vi "Git-Enterprise-Get All Repos In Org.vi"(8 "Error In":errorcluster, 9 "Organization":string, 10 "Server":string, 11 "Refnum in":T2) -> (0 "Error out":errorcluster, 3 "Repos":T1[](array[typedef]))   [LabVIEW 2020]
uses:
  <vilib>/httpClient/ClientHandle.ctl
  Git-Repo JSON Typedef.ctl
  <vilib>/JDP Science/JSONtext/String Subset.vi
  <vilib>/JDP Science/JSONtext/Parsing/Parse Full Path or Item Name.vi
  <vilib>/JDP Science/JSONtext/Offset/Find Item Locations by Path.vi
  <vilib>/httpClient/LabVIEWHTTPClient.lvlib
  <vilib>/JDP Science/JSONtext/JSONtext.lvlib
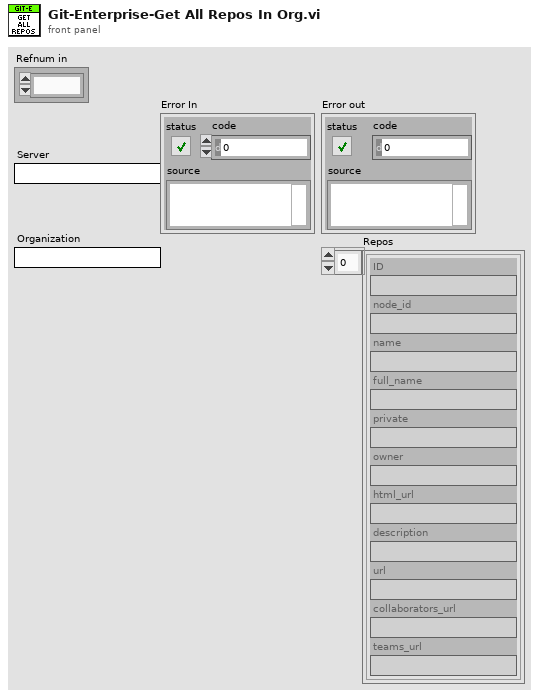
[diagram p1: front panel]
types:
  T1 = typedef "Git-Repo JSON Typedef.ctl" = cluster{"ID":string, "node_id":string, "name":string, "full_name":string, "private":string, "owner":string, "html_url":string, "description":string, "url":string, "collaborators_url":string, "teams_url":string}
  T2 = typedef "LabVIEWHTTPClient.lvlib/ClientHandle.ctl" = refnum<k1>
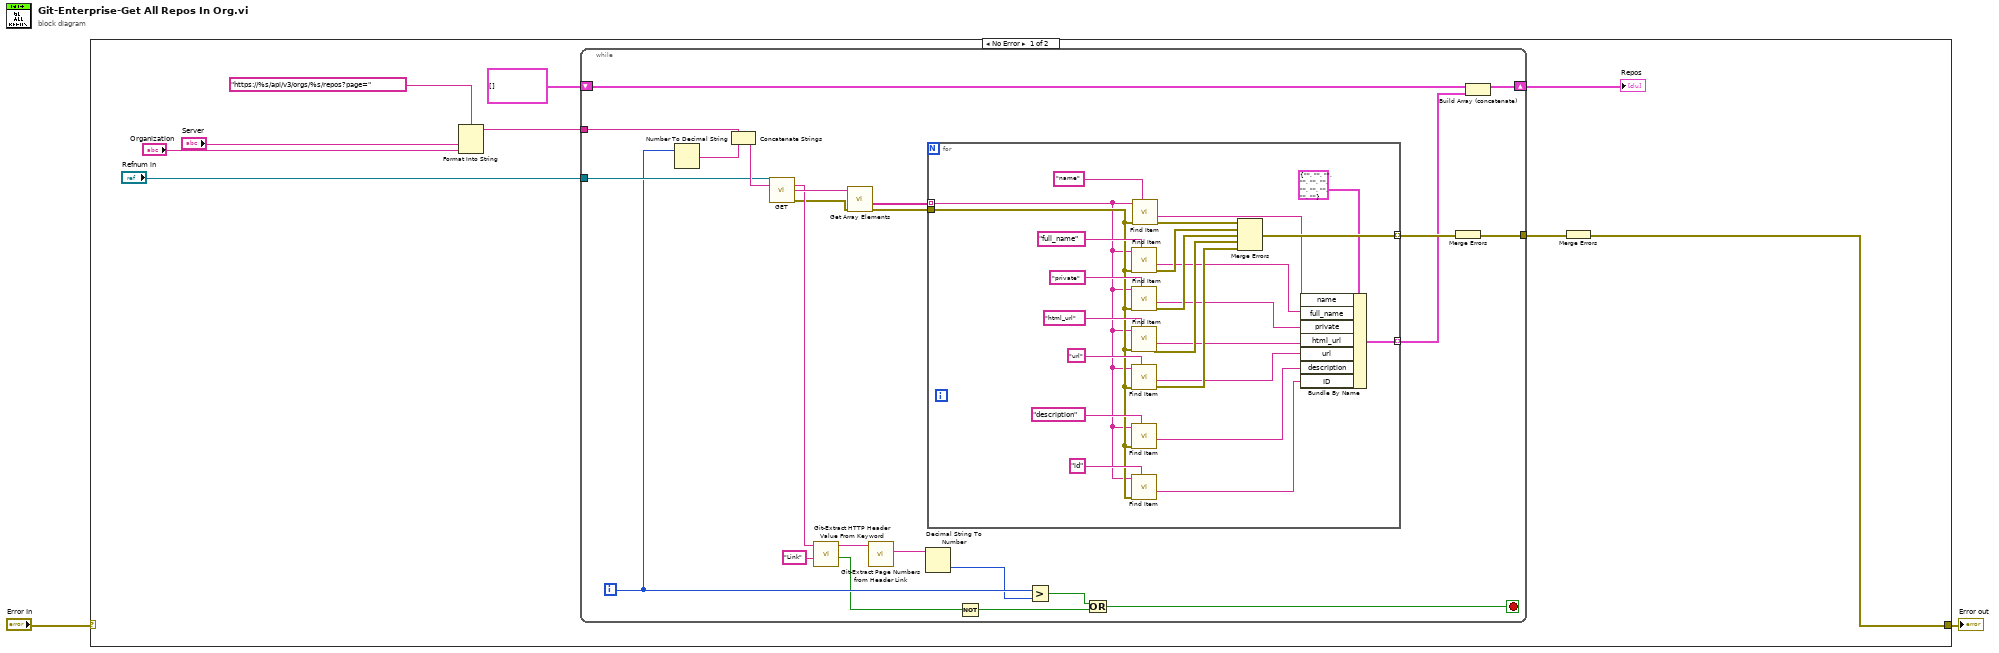
[diagram p0: block diagram]
diagram:
  n1 = case shown="No Error" "Error In" {
    selector: "Error In" -> [_ w59]
    tunnel: [w4 w59] -> w1
    frame No Error {
      n2 = Format Into String(format string="https://%s/api/v3/orgs/%s/repos?page=" ("url"), "Server", "Organization") -> (resulting string=w11:string)  [unwired: 2 in, 1 out]
      n3 = while {
        tunnel: "Refnum in" -> [w33]
        shift-right: [w29] -> w3
        shift-left: T1[] [] -> [w30]
        tunnel: w11 -> [w20]
        tunnel: [w18] -> w5
        i -> [w32]
        stop <- w13 stop-if-true
        n4 = Number To Decimal String(number=w32) -> (decimal integer string=w31:string)  [unwired: 1 in]
        n5 = Concatenate Strings(w20, w31) -> (w34:string)
        n6 = call <vilib>:"GET.vi"("client handle"=w33, "url"=w34) -> ("headers"=w22:string, "body"=w26:string, "error out"=w17:errorcluster)  [unwired: 10 in, 1 out]
        n7 = call "Git-Extract HTTP Header Value From Keyword.vi"("Key"="Link", "Header Info"=w22) -> ("Found"=w15:bool, "Value"=w23:string)  [unwired: 8 in]
        n8 = call <vilib>:"Get Array Elements.vi"("error in (no error)"=w17, "JSON"=w26) -> ("error out"=w28:errorcluster, "<JSON>"=w27:string[])  [unwired: 7 in, 1 out]
        n9 = call "Git-Extract Page Numbers from Header Link.vi"("Link"=w23) -> ("Pages"=w25:string)  [unwired: 9 in, 1 out]
        n10 = Decimal String To Number(string=w25) -> (number=w21:i32)  [unwired: 2 in, 1 out]
        n11 = for {
          tunnel: w27 -> [w36] mode=indexing
          tunnel: w28 -> [w37]
          tunnel: [w48] -> w19 mode=indexing
          tunnel: [w39] -> w12 mode=indexing
          n12 = call <vilib>:"Find Item.vi"("$Path or Item Name"="full_name", "error in (no error)"=w37, "JSON"=w36) -> ("error out"=w52:errorcluster, "<JSON>"=w45:string)  [unwired: 5 in, 2 out]
          n13 = call <vilib>:"Find Item.vi"("$Path or Item Name"="private", "error in (no error)"=w37, "JSON"=w36) -> ("error out"=w51:errorcluster, "<JSON>"=w44:string)  [unwired: 5 in, 2 out]
          n14 = call <vilib>:"Find Item.vi"("$Path or Item Name"="html_url", "error in (no error)"=w37, "JSON"=w36) -> ("error out"=w50:errorcluster, "<JSON>"=w43:string)  [unwired: 5 in, 2 out]
          n15 = call <vilib>:"Find Item.vi"("$Path or Item Name"="url", "error in (no error)"=w37, "JSON"=w36) -> ("error out"=w49:errorcluster, "<JSON>"=w42:string)  [unwired: 5 in, 2 out]
          n16 = call <vilib>:"Find Item.vi"("$Path or Item Name"="description", "error in (no error)"=w37, "JSON"=w36) -> ("<JSON>"=w40:string)  [unwired: 5 in, 3 out]
          n17 = call <vilib>:"Find Item.vi"("$Path or Item Name"="id", "error in (no error)"=w37, "JSON"=w36) -> ("<JSON>"=w35:string)  [unwired: 5 in, 3 out]
          n18 = call <vilib>:"Find Item.vi"("$Path or Item Name"="name", "error in (no error)"=w37, "JSON"=w36) -> ("error out"=w53:errorcluster, "<JSON>"=w46:string)  [unwired: 5 in, 2 out]
          n19 = Merge Errors(w53, w52, w51, w50, w49) -> (w48:errorcluster)
          n20 = Bundle By Name(cluster=T1 {"ID"="", "node_id"="", "name"="", "full_name"="", "private"="", "owner"="", "html_url"="", "description"="", "url"="", "collaborators_url"="", "teams_url"=""} ("Cluster"), "name"=w46, "full_name"=w45, "private"=w44, "html_url"=w43, "url"=w42, "description"=w40, "ID"=w35) -> (w39:T1)
        }
        n21 = Not(x=w15) -> (.not. x?=w16:bool)
        n22 = Greater?(x=w32, y=w21) -> (0:w14:bool)
        n23 = Or(x=w14, y=w16) -> (x .or. y?=w13:bool)
        n24 = Merge Errors(w19) -> (w18:errorcluster)
        n25 = Build Array (concatenate)(w30, w12) -> (w29:T1[])
      }
      "Repos" <- w3
      n26 = Merge Errors(w5) -> (w4:errorcluster)
    }
    frame Error {
    }
  }
  "Error out" <- w1
